vi "osa_update display.vi"(9 "sensor LUT":variant, 10 "data":u32[](array[numeric]), 11 "display refnums in":T1) -> (3 "display refnums out":T1)   [LabVIEW 2021]
panel:
  # "OSA subVI: parse data and update display"
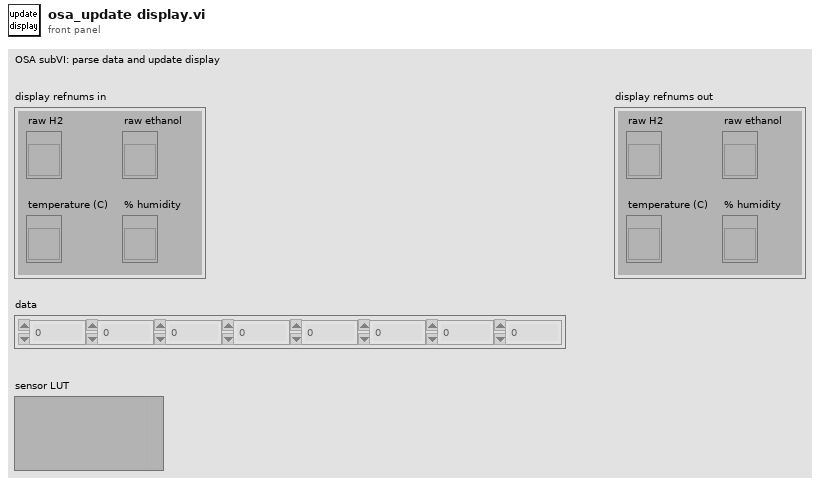
[diagram p1: front panel]
types:
  T1 = cluster{"raw H2":refnum<vi>, "raw ethanol":refnum<vi>, "temperature (C)":refnum<vi>, "% humidity":refnum<vi>}
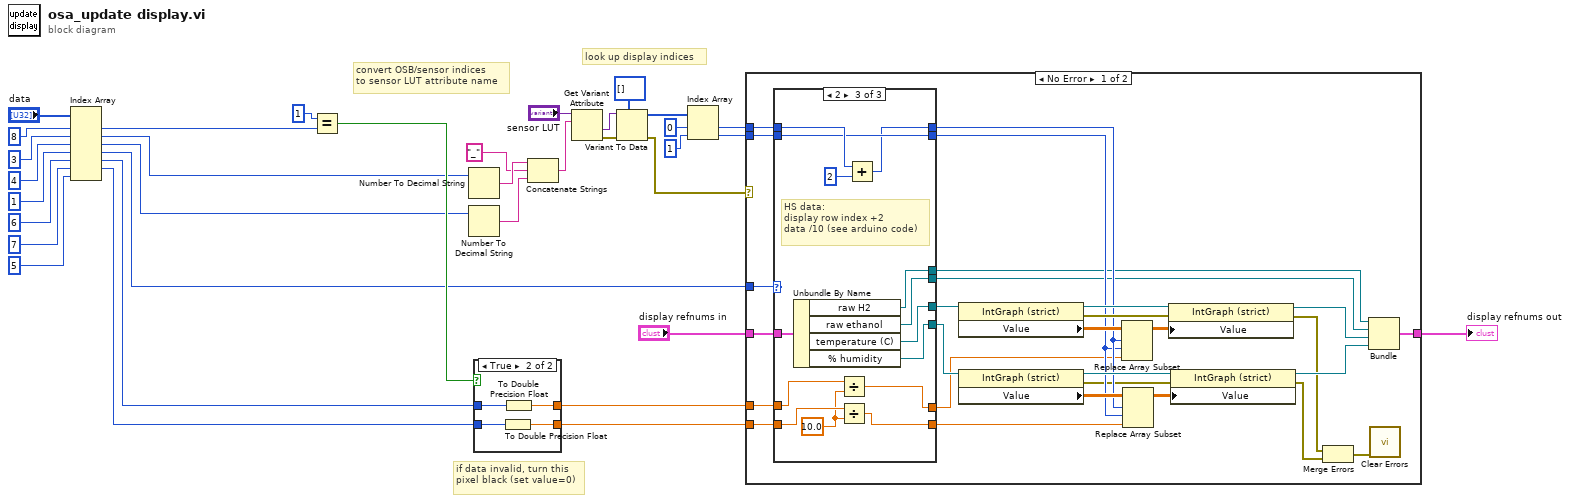
[diagram p0: block diagram]
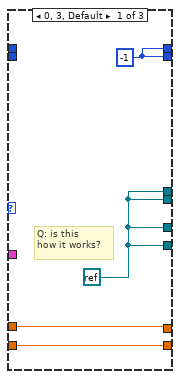
[diagram p2: hidden frame]
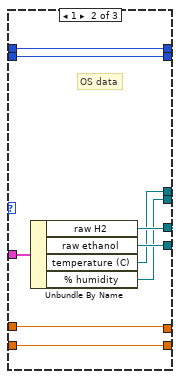
[diagram p3: hidden frame]
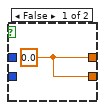
[diagram p5: hidden frame]
diagram:
  # "if data invalid, turn this pixel black (set value=0)"
  # "look up display indices"
  # "convert OSB/sensor indices\nto sensor LUT attribute name"
  n1 = Index Array(array="data", index #1=8, index #2=3, index #3=4, index #4=1, index #5=6, index #6=7, index #7=5) -> (element #1=w33:u32, element #2=w3:u32, element #3=w2:u32, element #4=w1:u32, element #5=w24:u32, element #6=w25:u32)  [unwired: 1 out]
  n2 = Equal?(x=u32 1, y=w33) -> (x = y?=w7:bool)
  n3 = Number To Decimal String(number=w3) -> (decimal integer string=w21:string)  [unwired: 1 in]
  n4 = Number To Decimal String(number=w2) -> (decimal integer string=w20:string)  [unwired: 1 in]
  n5 = case shown="True" w7 {
    tunnel: w25 -> [_ w39]
    tunnel: w24 -> [_ w38]
    tunnel: [w35 w37] -> w9
    tunnel: [w35 w36] -> w8
    frame False {
      w35 = 0.0
    }
    frame True {
      n6 = To Double Precision Float(number=w39) -> (double precision float=w36:dbl)
      n7 = To Double Precision Float(number=w38) -> (double precision float=w37:dbl)
    }
  }
  n8 = Concatenate Strings(w21, "_", w20) -> (w18:string)
  n9 = Get Variant Attribute(Variant="sensor LUT", name=w18) -> (value=w17:variant, error out=w6:errorcluster)  [unwired: 2 in, 2 out]
  n10 = Variant To Data(error in=w6, type=i32[] [], Variant=w17) -> (data=w13:i32[], error out=w5:errorcluster)
  n11 = Index Array(array=w13, index #1=0, index #2=1) -> (element #1=w11:i32, element #2=w10:i32)
  n12 = case shown="No Error" w5 {
    tunnel: w1 -> [w67 _]
    tunnel: "display refnums in" -> [w66 w95]
    tunnel: [w65 w95] -> w22
    tunnel: w11 -> [w58 _]
    tunnel: w10 -> [w57 _]
    tunnel: w9 -> [w43 _]
    tunnel: w8 -> [w42 _]
    frame No Error {
      n13 = case shown="2" w67 {
        tunnel: [w71 w79 w93] -> w56
        tunnel: [w71 w78 w92] -> w55
        tunnel: [w71 w76 w91] -> w50
        tunnel: [w71 w77 w90] -> w51
        tunnel: w66 -> [_ w80 w94]
        tunnel: w58 -> [_ w75 w88]
        tunnel: w57 -> [_ w74 w87]
        tunnel: [w70 w75 w86] -> w53
        tunnel: [w70 w74 w87] -> w52
        tunnel: [w69 w73 w82] -> w41
        tunnel: w43 -> [w69 w73 w85]
        tunnel: [w68 w72 w81] -> w40
        tunnel: w42 -> [w68 w72 w84]
        frame 0, 3, Default {
          w70 = -1
          w71 = refnum<k0> refnum
          # "Q: is this\nhow it works?"
        }
        frame 1 {
          # "OS data"
          n14 = Unbundle By Name(w80) -> ("raw H2"=w79:refnum<vi>, "raw ethanol"=w78:refnum<vi>, "temperature (C)"=w77:refnum<vi>, "% humidity"=w76:refnum<vi>)
        }
        frame 2 {
          w83 = 10.0 ("y")
          # "HS data:\ndisplay row index +2\ndata /10 (see arduino code)"
          n15 = Unbundle By Name(w94) -> ("raw H2"=w90:refnum<vi>, "raw ethanol"=w91:refnum<vi>, "temperature (C)"=w93:refnum<vi>, "% humidity"=w92:refnum<vi>)
          n16 = Divide(x=w85, y=w83) -> (x/y=w82:dbl)
          n17 = Divide(x=w84, y=w83) -> (x/y=w81:dbl)
          n18 = Add(x=w88, y=2) -> (x+y=w86:i32)
        }
      }
      n19 = property class="IntGraph (strict)"(reference=w56) -> (reference out=w62:refnum<vi>, error out=w54:errorcluster, "Value"=w64:dbl[][])  [unwired: 1 in]
      n20 = property class="IntGraph (strict)"(reference=w55) -> (reference out=w60:refnum<vi>, error out=w47:errorcluster, "Value"=w63:dbl[][])  [unwired: 1 in]
      n21 = Replace Array Subset(array=w64, new element=w41, index (row)=w53, index (col)=w52) -> (w61:dbl[][])
      n22 = Replace Array Subset(array=w63, new element=w40, index (row)=w53, index (col)=w52) -> (w59:dbl[][])
      n23 = property class="IntGraph (strict)"(reference=w62, error in=w54, "Value"=w61) -> (reference out=w49:refnum<vi>, error out=w45:errorcluster)
      n24 = property class="IntGraph (strict)"(reference=w60, error in=w47, "Value"=w59) -> (reference out=w48:refnum<vi>, error out=w44:errorcluster)
      n25 = Merge Errors(w45, w44) -> (w46:errorcluster)
      n26 = Bundle("raw H2"=w51, "raw ethanol"=w50, "temperature (C)"=w49, "% humidity"=w48) -> (w65:T1)  [unwired: 1 in]
      n27 = call <vilib>:"Clear Errors.vi"("error in (no error)"=w46) -> ()  [unwired: 5 in, 2 out]
    }
    frame Error {
      # "if anything unexpected happens,\ndon't update display at all"
    }
  }
  "display refnums out" <- w22
